vi "Save TDMS.vi"(8 "error in (no error)":errorcluster, 10 "Save Format":u16(ring) items=["TXT", "TDMS"], 11 "Binary counter in":refnum<class "Binary counter.lvclass">) -> (0 "error out":errorcluster, 3 "Binary counter out":refnum<class "Binary counter.lvclass">)   [LabVIEW 2020, in "Binary counter.lvlib" / "Binary counter.lvclass"]
uses:
  Binary counter.lvclass
  C:/Program Files/National Instruments/LabVIEW 2020/vi.lib/ActorFramework/Actor/Actor.lvclass
  Login bin/Login bin/Login bin.lvclass
  TDMS contador/TDMS contador/TDMS contador.lvclass
  C:/Users/Ceci Saldivar/Desktop/ceci/7mo semestre/Henry/Actor-Tarea-10-12-2020/Login bin/Login bin/Login bin.lvclass
  Binary counter.lvclass/Binary counter.ctl
  <vilib>/ActorFramework/Actor/Actor.lvclass
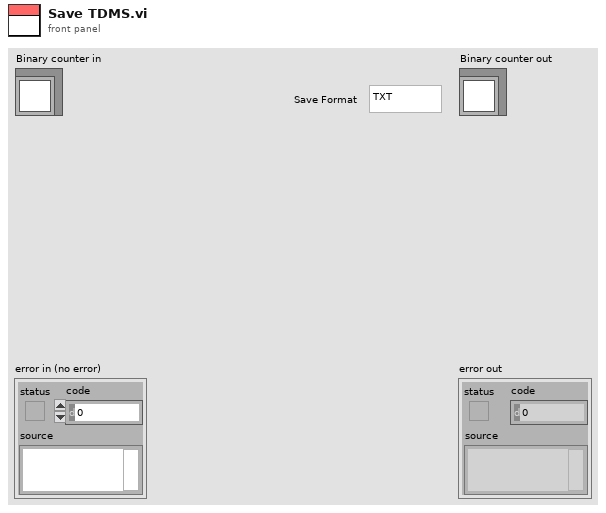
[diagram p1: front panel]
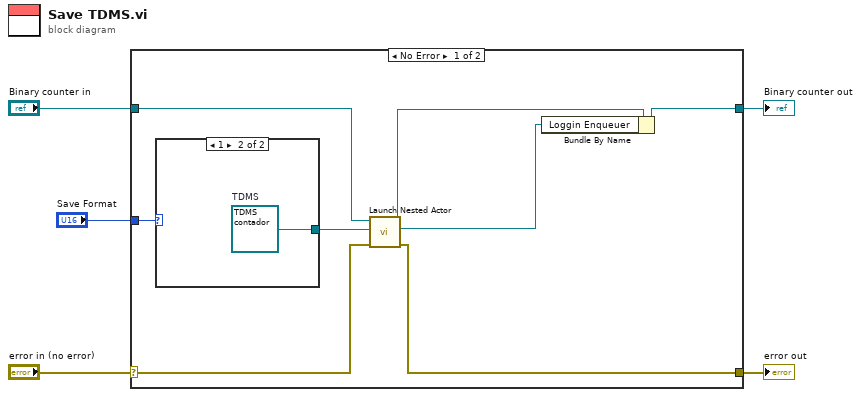
[diagram p0: block diagram]
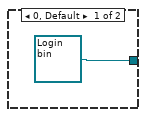
[diagram p2: hidden frame]
diagram:
  n1 = case shown="No Error" "error in (no error)" {
    selector: "error in (no error)" -> [w9 w17]
    tunnel: [w8 w17] -> w4
    tunnel: [w13 w16] -> w2
    tunnel: "Binary counter in" -> [w11 w16]
    tunnel: "Save Format" -> [w12 _]
    frame No Error {
      n2 = case shown="1" w12 {
        tunnel: [refnum<class "Login bin.lvclass"> refnum ("Login bin.lvlib:Login bin.lvclass") w15] -> w10
        frame 0, Default {
        }
        frame 1 {
          w15 = refnum<class "TDMS contador.lvclass"> refnum  # TDMS
        }
      }
      n3 = call <vilib>:"Launch Nested Actor.vi"("error in (no error)"=w9, "Nested Actor"=w10, "Caller Actor in"=w11) -> ("error out"=w8:errorcluster, "Nested Actor's Enqueuer"=w6:refnum<class "Message Enqueuer.lvclass">, "Caller Actor out"=w7:refnum<class "Binary counter.lvclass">)  [unwired: 6 in]
      n4 = Bundle By Name(cluster=w7, "Loggin Enqueuer"=w6) -> (w13:refnum<class "Binary counter.lvclass">)
    }
    frame Error {
    }
  }
  "error out" <- w4
  "Binary counter out" <- w2
